vi "SBCoolingOperationWindow.vi"() -> ()   [LabVIEW 2019]
panel:
  in  "Total time [ms] :":dbl
  in  "quit":bool
  in  "save times":bool
  in  "load params":bool
  in  "Average motional state :":dbl
  in  "Maximum n levels :":dbl
  in  "Carrier Rabi Frequency :":dbl
  in  "Lamb-Dicke Parameter :":dbl
  in  "show times":bool
  in  "sb time array":dbl[](array[numeric]) caption="Sideband Cooling Times"
  # "Parameters :"
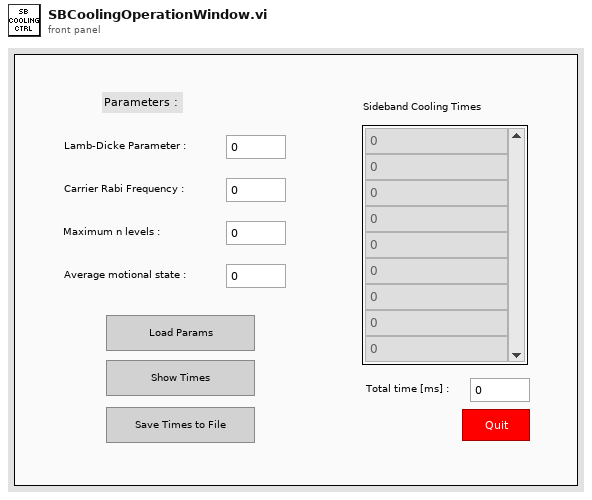
[diagram p1: front panel]
types:
  T1 = cluster{"nlevels":i32, "nbar":dbl, "eta":dbl, "omega":dbl, "save":dbl}
  T2 = cluster{"nlevels":i32, "nbar":dbl, "eta":dbl, "omega":dbl, "save":i32}
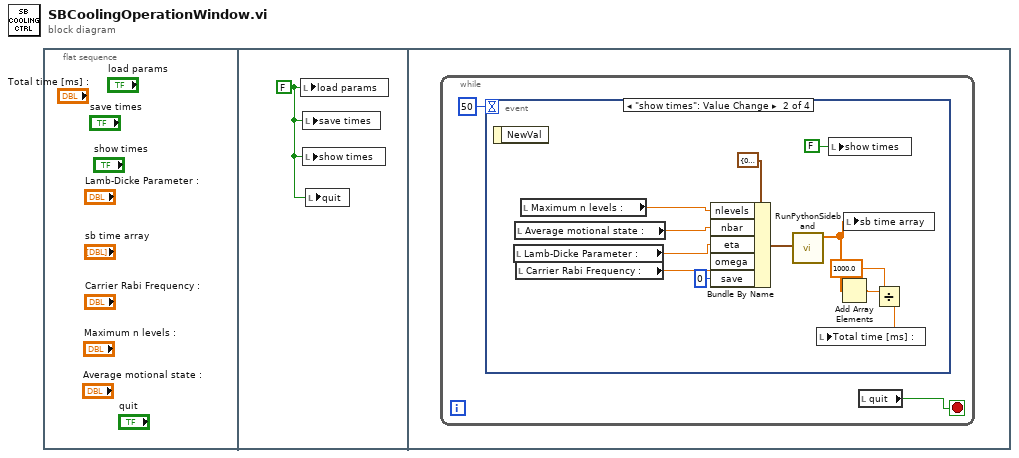
[diagram p0: block diagram]
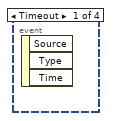
[diagram p2: hidden frame]
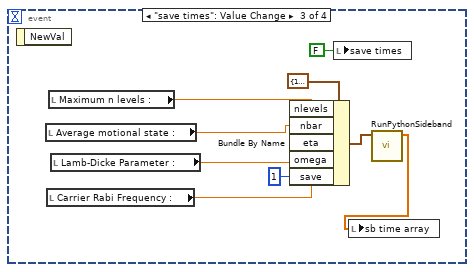
[diagram p3: hidden frame]
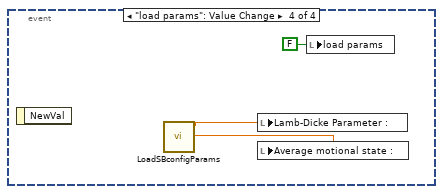
[diagram p4: hidden frame]
diagram:
  n1 = flat-sequence {
    frame #0 {
    }
    frame #1 {
      w1 = FALSE ("load params")
      n2 = local write "load params"(w1) -> ()
      n3 = local write "save times"(w1) -> ()
      n4 = local write "show times"(w1) -> ()
      n5 = local write "quit"(w1) -> ()
    }
    frame #2 {
      n6 = while {
        stop <- w2 stop-if-true
        n7 = event shown="[1] \"show times\": Value Change" {
          selector: _ -> [_ _ _ _]
          dyn-events: _ -> [_ _ _ _]
          timeout: 50 -> [_ _ _ _]
          event Timeout {
            n8 = event-data() -> ()  [unwired: 1 in, 3 out]
          }
          event "show times": Value Change {
            n9 = event-data() -> ()  [unwired: 1 in, 1 out]
            n10 = local read "Lamb-Dicke Parameter :"() -> (w13:dbl)
            n11 = local read "Average motional state :"() -> (w14:dbl)
            n12 = local read "Carrier Rabi Frequency :"() -> (w12:dbl)
            n13 = local read "Maximum n levels :"() -> (w15:dbl)
            n14 = Bundle By Name(cluster=T1 {"nlevels"=0, "nbar"=0.0, "eta"=0.0, "omega"=0.0, "save"=0.0} ("params in"), "nlevels"=w15, "nbar"=w14, "eta"=w13, "omega"=w12, "save"=0) -> (w8:T1)
            n15 = call "RunPythonSideband.vi"("params in"=w8) -> ("times array out"=w7:dbl[])  [unwired: 9 in, 1 out]
            n16 = local write "show times"(FALSE ("show times")) -> ()
            n17 = Add Array Elements(numeric array=w7) -> (sum=w6:dbl)
            n18 = local write "sb time array"(w7) -> ()
            n19 = Divide(x=w6, y=1000.0) -> (x/y=w4:dbl)
            n20 = local write "Total time [ms] :"(w4) -> ()
          }
          event "save times": Value Change {
            n21 = event-data() -> ()  [unwired: 1 in, 1 out]
            n22 = local read "Average motional state :"() -> (w21:dbl)
            n23 = local read "Carrier Rabi Frequency :"() -> (w19:dbl)
            n24 = local read "Maximum n levels :"() -> (w22:dbl)
            n25 = local read "Lamb-Dicke Parameter :"() -> (w20:dbl)
            n26 = Bundle By Name(cluster=T2 {"nlevels"=1000, "nbar"=57.0, "eta"=0.0066, "omega"=215.0, "save"=0} ("params in"), "nlevels"=w22, "nbar"=w21, "eta"=w20, "omega"=w19, "save"=1) -> (w23:T2)
            n27 = local write "save times"(FALSE ("save times")) -> ()
            n28 = call "RunPythonSideband.vi"("params in"=w23) -> ("times array out"=w17:dbl[])  [unwired: 9 in, 1 out]
            n29 = local write "sb time array"(w17) -> ()
          }
          event "load params": Value Change {
            n30 = event-data() -> ()  [unwired: 1 in, 1 out]
            n31 = call "LoadSBconfigParams.vi"() -> ("nbar"=w25:dbl, "eta"=w26:dbl)  [unwired: 9 in, 1 out]
            n32 = local write "Lamb-Dicke Parameter :"(w26) -> ()
            n33 = local write "Average motional state :"(w25) -> ()
            n34 = local write "load params"(FALSE ("load params")) -> ()
          }
        }
        n35 = local read "quit"() -> (w2:bool)
      }
    }
  }
